vi "Calculate Checksum.vi"(7 "Message In":T1, 11 "Error In":errorcluster) -> (8 "Message Out":T1, 10 "Checksum":string, 15 "Error Out":errorcluster)   [LabVIEW 2023, in "ICanCommunicate.lvclass"]
doc: "Completes a message by calculating checksum and appending it to the message."
uses:
  Message.ctl
  <vilib>/security/Message Digest/API/Instances/Byte Array/SHA-256 Byte Array Checksum.vi
  ICanCommunicate.lvclass
  <vilib>/security/Message Digest/API/NI_Message Digest API.lvlib
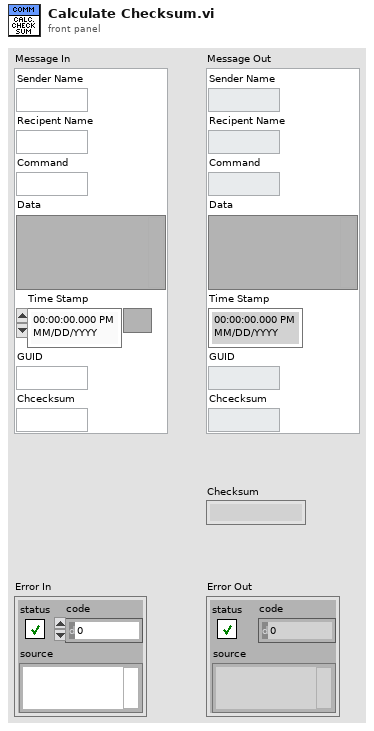
[diagram p1: front panel]
types:
  T1 = typedef "ICanCommunicate.lvclass/Message.ctl" = cluster{"Sender Name":string, "Recipent Name":string, "Command":string, "Data":variant, "Time Stamp":timestamp, "GUID":string, "Chcecksum":string}
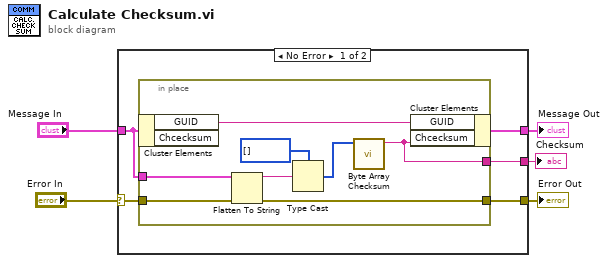
[diagram p0: block diagram]
diagram:
  n1 = case shown="No Error" "Error In" {
    selector: "Error In" -> [w10 w19]
    tunnel: [w9 w19] -> w4
    tunnel: "Message In" -> [w8 _]
    tunnel: [w7 _] -> w2
    tunnel: [w6 _] -> w1
    frame No Error {
      n2 = in-place {
        in-place-border: w10 -> [w15]
        in-place-border: [w14] -> w9
        in-place-border: w8 -> [w13]
        in-place-border: [w11] -> w6
        n3 = in-place-cluster #1(w8) -> ("GUID"=w12:string)  [unwired: 1 out]
        n4 = Flatten To String(anything=w13, error in (no error)=w15) -> (data string=w17:string, error out=w14:errorcluster)  [unwired: 2 in, 1 out]
        n5 = Type Cast(type=u8[] [], x=w17) -> (*(type *) &x=w16:u8[])
        n6 = call-poly <vilib>:"Byte Array Checksum.vi"("buffer"=w16) -> ("digest"=w11:string)  [unwired: 10 in]
        n7 = in-place-cluster #1("GUID"=w12, "Chcecksum"=w11) -> (w7:T1)
      }
    }
    frame Error {
    }
  }
  "Error Out" <- w4
  "Message Out" <- w2
  "Checksum" <- w1
